vi "updateValues.vi"(8 "error in (no error)":errorcluster, 9 "channel index":i32, 10 "NumberDO":i32, 11 "NumberDI":i32) -> (0 "error out":errorcluster)   [LabVIEW 2020, in "Productivity1000PLC.lvclass"]
uses:
  Productivity1000PLC.lvclass
  shared/OnOffTypeDef.ctl
  shared/CompressAndUpdate(Poly)/CompressAndUpdate(Enum).vi
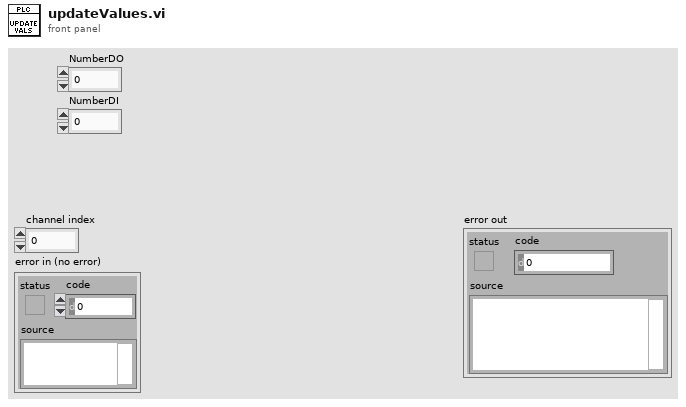
[diagram p1: front panel]
types:
  T1 = typedef "OnOffTypeDef.ctl" = enum16{"off", "on"}
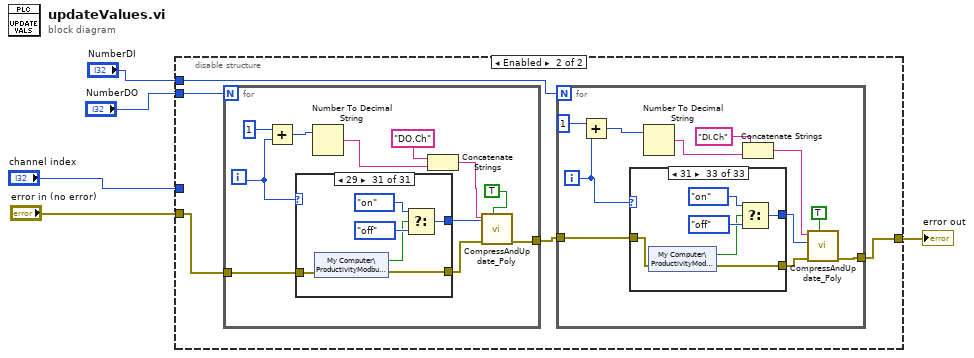
[diagram p0: block diagram]
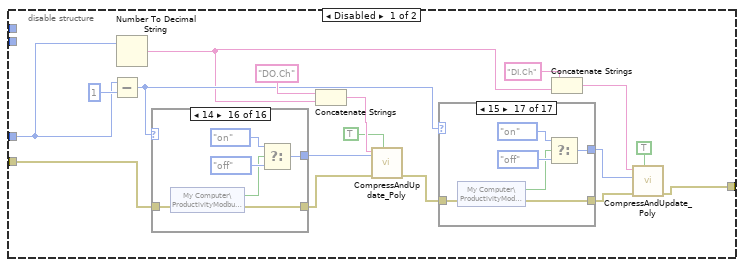
[diagram p2: hidden frame]
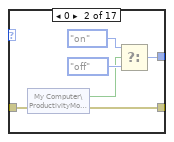
[diagram p4: hidden frame]
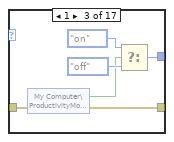
[diagram p5: hidden frame]
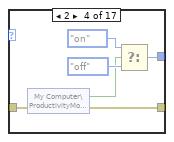
[diagram p6: hidden frame]
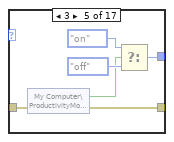
[diagram p7: hidden frame]
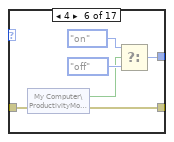
[diagram p8: hidden frame]
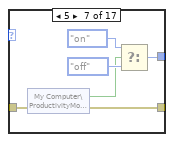
[diagram p9: hidden frame]
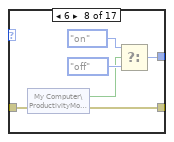
[diagram p10: hidden frame]
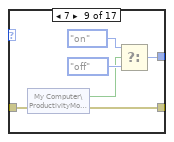
[diagram p11: hidden frame]
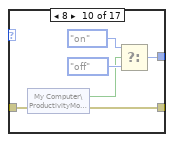
[diagram p12: hidden frame]
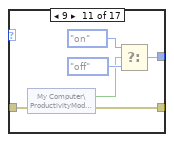
[diagram p13: hidden frame]
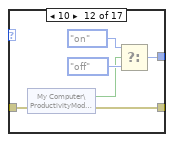
[diagram p14: hidden frame]
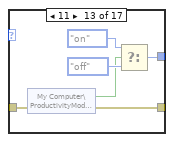
[diagram p15: hidden frame]
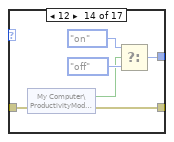
[diagram p16: hidden frame]
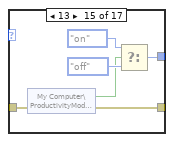
[diagram p17: hidden frame]
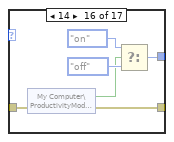
[diagram p18: hidden frame]
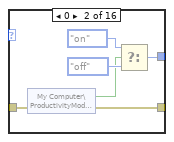
[diagram p20: hidden frame]
diagram:
  n1 = disable-structure shown="Enabled" {
    disable-tunnel: [w15 w213] -> w5
    disable-tunnel: "channel index" -> [w14 _]
    disable-tunnel: "error in (no error)" -> [w13 w215]
    disable-tunnel: "NumberDO" -> [_ w212]
    disable-tunnel: "NumberDI" -> [_ w211]
    frame Disabled {
      n2 = Subtract(x=w14, y=1) -> (x-y=w10:i32)
      n3 = Number To Decimal String(number=w14) -> (decimal integer string=w6:string)  [unwired: 1 in]
      n4 = case shown="14" w10 {
        tunnel: w13 -> [w120 w121 w127 w133 w139 w145 w151 w157 w163 w169 w175 w181 w187 w193 w199 w205]
        tunnel: [w120 w123 w129 w135 w141 w147 w153 w159 w165 w171 w177 w183 w189 w195 w201 w207] -> w9
        tunnel: [_ w122 w128 w134 w140 w146 w152 w158 w164 w170 w176 w182 w188 w194 w200 w206] -> w12
        frame Default {
        }
        frame 0 {
          n5 = shared-variable "My Computer\\ProductivityModbus.lvlib\\DO1"(error in=w121) -> (w124:bool, error out=w123:errorcluster)
          n6 = Select(t=OnOffTypeDef."on" ("Channel 0"), s=w124, f=OnOffTypeDef."off" ("Channel 0")) -> (s? t:f=w122:T1)
        }
        frame 1 {
          n7 = shared-variable "My Computer\\ProductivityModbus.lvlib\\DO2"(error in=w127) -> (w130:bool, error out=w129:errorcluster)
          n8 = Select(t=OnOffTypeDef."on" ("Channel 0"), s=w130, f=OnOffTypeDef."off" ("Channel 0")) -> (s? t:f=w128:T1)
        }
        frame 2 {
          n9 = shared-variable "My Computer\\ProductivityModbus.lvlib\\DO3"(error in=w133) -> (w136:bool, error out=w135:errorcluster)
          n10 = Select(t=OnOffTypeDef."on" ("Channel 0"), s=w136, f=OnOffTypeDef."off" ("Channel 0")) -> (s? t:f=w134:T1)
        }
        frame 3 {
          n11 = shared-variable "My Computer\\ProductivityModbus.lvlib\\DO4"(error in=w139) -> (w142:bool, error out=w141:errorcluster)
          n12 = Select(t=OnOffTypeDef."on" ("Channel 0"), s=w142, f=OnOffTypeDef."off" ("Channel 0")) -> (s? t:f=w140:T1)
        }
        frame 4 {
          n13 = shared-variable "My Computer\\ProductivityModbus.lvlib\\DO5"(error in=w145) -> (w148:bool, error out=w147:errorcluster)
          n14 = Select(t=OnOffTypeDef."on" ("Channel 0"), s=w148, f=OnOffTypeDef."off" ("Channel 0")) -> (s? t:f=w146:T1)
        }
        frame 5 {
          n15 = shared-variable "My Computer\\ProductivityModbus.lvlib\\DO6"(error in=w151) -> (w154:bool, error out=w153:errorcluster)
          n16 = Select(t=OnOffTypeDef."on" ("Channel 0"), s=w154, f=OnOffTypeDef."off" ("Channel 0")) -> (s? t:f=w152:T1)
        }
        frame 6 {
          n17 = shared-variable "My Computer\\ProductivityModbus.lvlib\\DO7"(error in=w157) -> (w160:bool, error out=w159:errorcluster)
          n18 = Select(t=OnOffTypeDef."on" ("Channel 0"), s=w160, f=OnOffTypeDef."off" ("Channel 0")) -> (s? t:f=w158:T1)
        }
        frame 7 {
          n19 = shared-variable "My Computer\\ProductivityModbus.lvlib\\DO8"(error in=w163) -> (w166:bool, error out=w165:errorcluster)
          n20 = Select(t=OnOffTypeDef."on" ("Channel 0"), s=w166, f=OnOffTypeDef."off" ("Channel 0")) -> (s? t:f=w164:T1)
        }
        frame 8 {
          n21 = shared-variable "My Computer\\ProductivityModbus.lvlib\\DO9"(error in=w169) -> (w172:bool, error out=w171:errorcluster)
          n22 = Select(t=OnOffTypeDef."on" ("Channel 0"), s=w172, f=OnOffTypeDef."off" ("Channel 0")) -> (s? t:f=w170:T1)
        }
        frame 9 {
          n23 = shared-variable "My Computer\\ProductivityModbus.lvlib\\DO10"(error in=w175) -> (w178:bool, error out=w177:errorcluster)
          n24 = Select(t=OnOffTypeDef."on" ("Channel 0"), s=w178, f=OnOffTypeDef."off" ("Channel 0")) -> (s? t:f=w176:T1)
        }
        frame 10 {
          n25 = shared-variable "My Computer\\ProductivityModbus.lvlib\\DO11"(error in=w181) -> (w184:bool, error out=w183:errorcluster)
          n26 = Select(t=OnOffTypeDef."on" ("Channel 0"), s=w184, f=OnOffTypeDef."off" ("Channel 0")) -> (s? t:f=w182:T1)
        }
        frame 11 {
          n27 = shared-variable "My Computer\\ProductivityModbus.lvlib\\DO12"(error in=w187) -> (w190:bool, error out=w189:errorcluster)
          n28 = Select(t=OnOffTypeDef."on" ("Channel 0"), s=w190, f=OnOffTypeDef."off" ("Channel 0")) -> (s? t:f=w188:T1)
        }
        frame 12 {
          n29 = shared-variable "My Computer\\ProductivityModbus.lvlib\\DO13"(error in=w193) -> (w196:bool, error out=w195:errorcluster)
          n30 = Select(t=OnOffTypeDef."on" ("Channel 0"), s=w196, f=OnOffTypeDef."off" ("Channel 0")) -> (s? t:f=w194:T1)
        }
        frame 13 {
          n31 = shared-variable "My Computer\\ProductivityModbus.lvlib\\DO14"(error in=w199) -> (w202:bool, error out=w201:errorcluster)
          n32 = Select(t=OnOffTypeDef."on" ("Channel 0"), s=w202, f=OnOffTypeDef."off" ("Channel 0")) -> (s? t:f=w200:T1)
        }
        frame 14 {
          n33 = shared-variable "My Computer\\ProductivityModbus.lvlib\\DO15"(error in=w205) -> (w208:bool, error out=w207:errorcluster)
          n34 = Select(t=OnOffTypeDef."on" ("Channel 0"), s=w208, f=OnOffTypeDef."off" ("Channel 0")) -> (s? t:f=w206:T1)
        }
      }
      n35 = Concatenate Strings("DO.Ch" ("command or variable name"), w6) -> (w22:string)
      n36 = call-poly "CompressAndUpdate_Poly.vi"("force CVT update (false)"=TRUE, "error in"=w9, "enum variant"=w12, "command or variable name"=w22) -> ("error out"=w8:errorcluster)  [unwired: 7 in]
      n37 = case shown="15" w10 {
        tunnel: w8 -> [w23 w24 w30 w36 w42 w48 w54 w60 w66 w72 w78 w84 w90 w96 w102 w108 w114]
        tunnel: [w23 w26 w32 w38 w44 w50 w56 w62 w68 w74 w80 w86 w92 w98 w104 w110 w116] -> w7
        tunnel: [_ w25 w31 w37 w43 w49 w55 w61 w67 w73 w79 w85 w91 w97 w103 w109 w115] -> w11
        frame Default {
        }
        frame 0 {
          n38 = shared-variable "My Computer\\ProductivityModbus.lvlib\\DI1"(error in=w24) -> (w27:bool, error out=w26:errorcluster)
          n39 = Select(t=OnOffTypeDef."on" ("Channel 0"), s=w27, f=OnOffTypeDef."off" ("Channel 0")) -> (s? t:f=w25:T1)
        }
        frame 1 {
          n40 = shared-variable "My Computer\\ProductivityModbus.lvlib\\DI2"(error in=w30) -> (w33:bool, error out=w32:errorcluster)
          n41 = Select(t=OnOffTypeDef."on" ("Channel 0"), s=w33, f=OnOffTypeDef."off" ("Channel 0")) -> (s? t:f=w31:T1)
        }
        frame 2 {
          n42 = shared-variable "My Computer\\ProductivityModbus.lvlib\\DI3"(error in=w36) -> (w39:bool, error out=w38:errorcluster)
          n43 = Select(t=OnOffTypeDef."on" ("Channel 0"), s=w39, f=OnOffTypeDef."off" ("Channel 0")) -> (s? t:f=w37:T1)
        }
        frame 3 {
          n44 = shared-variable "My Computer\\ProductivityModbus.lvlib\\DI4"(error in=w42) -> (w45:bool, error out=w44:errorcluster)
          n45 = Select(t=OnOffTypeDef."on" ("Channel 0"), s=w45, f=OnOffTypeDef."off" ("Channel 0")) -> (s? t:f=w43:T1)
        }
        frame 4 {
          n46 = shared-variable "My Computer\\ProductivityModbus.lvlib\\DI5"(error in=w48) -> (w51:bool, error out=w50:errorcluster)
          n47 = Select(t=OnOffTypeDef."on" ("Channel 0"), s=w51, f=OnOffTypeDef."off" ("Channel 0")) -> (s? t:f=w49:T1)
        }
        frame 5 {
          n48 = shared-variable "My Computer\\ProductivityModbus.lvlib\\DI6"(error in=w54) -> (w57:bool, error out=w56:errorcluster)
          n49 = Select(t=OnOffTypeDef."on" ("Channel 0"), s=w57, f=OnOffTypeDef."off" ("Channel 0")) -> (s? t:f=w55:T1)
        }
        frame 6 {
          n50 = shared-variable "My Computer\\ProductivityModbus.lvlib\\DI7"(error in=w60) -> (w63:bool, error out=w62:errorcluster)
          n51 = Select(t=OnOffTypeDef."on" ("Channel 0"), s=w63, f=OnOffTypeDef."off" ("Channel 0")) -> (s? t:f=w61:T1)
        }
        frame 7 {
          n52 = shared-variable "My Computer\\ProductivityModbus.lvlib\\DI8"(error in=w66) -> (w69:bool, error out=w68:errorcluster)
          n53 = Select(t=OnOffTypeDef."on" ("Channel 0"), s=w69, f=OnOffTypeDef."off" ("Channel 0")) -> (s? t:f=w67:T1)
        }
        frame 8 {
          n54 = shared-variable "My Computer\\ProductivityModbus.lvlib\\DI9"(error in=w72) -> (w75:bool, error out=w74:errorcluster)
          n55 = Select(t=OnOffTypeDef."on" ("Channel 0"), s=w75, f=OnOffTypeDef."off" ("Channel 0")) -> (s? t:f=w73:T1)
        }
        frame 9 {
          n56 = shared-variable "My Computer\\ProductivityModbus.lvlib\\DI10"(error in=w78) -> (w81:bool, error out=w80:errorcluster)
          n57 = Select(t=OnOffTypeDef."on" ("Channel 0"), s=w81, f=OnOffTypeDef."off" ("Channel 0")) -> (s? t:f=w79:T1)
        }
        frame 10 {
          n58 = shared-variable "My Computer\\ProductivityModbus.lvlib\\DI11"(error in=w84) -> (w87:bool, error out=w86:errorcluster)
          n59 = Select(t=OnOffTypeDef."on" ("Channel 0"), s=w87, f=OnOffTypeDef."off" ("Channel 0")) -> (s? t:f=w85:T1)
        }
        frame 11 {
          n60 = shared-variable "My Computer\\ProductivityModbus.lvlib\\DI12"(error in=w90) -> (w93:bool, error out=w92:errorcluster)
          n61 = Select(t=OnOffTypeDef."on" ("Channel 0"), s=w93, f=OnOffTypeDef."off" ("Channel 0")) -> (s? t:f=w91:T1)
        }
        frame 12 {
          n62 = shared-variable "My Computer\\ProductivityModbus.lvlib\\DI13"(error in=w96) -> (w99:bool, error out=w98:errorcluster)
          n63 = Select(t=OnOffTypeDef."on" ("Channel 0"), s=w99, f=OnOffTypeDef."off" ("Channel 0")) -> (s? t:f=w97:T1)
        }
        frame 13 {
          n64 = shared-variable "My Computer\\ProductivityModbus.lvlib\\DI14"(error in=w102) -> (w105:bool, error out=w104:errorcluster)
          n65 = Select(t=OnOffTypeDef."on" ("Channel 0"), s=w105, f=OnOffTypeDef."off" ("Channel 0")) -> (s? t:f=w103:T1)
        }
        frame 14 {
          n66 = shared-variable "My Computer\\ProductivityModbus.lvlib\\DI15"(error in=w108) -> (w111:bool, error out=w110:errorcluster)
          n67 = Select(t=OnOffTypeDef."on" ("Channel 0"), s=w111, f=OnOffTypeDef."off" ("Channel 0")) -> (s? t:f=w109:T1)
        }
        frame 15 {
          n68 = shared-variable "My Computer\\ProductivityModbus.lvlib\\DI16"(error in=w114) -> (w117:bool, error out=w116:errorcluster)
          n69 = Select(t=OnOffTypeDef."on" ("Channel 0"), s=w117, f=OnOffTypeDef."off" ("Channel 0")) -> (s? t:f=w115:T1)
        }
      }
      n70 = Concatenate Strings("DI.Ch" ("command or variable name"), w6) -> (w18:string)
      n71 = call-poly "CompressAndUpdate_Poly.vi"("force CVT update (false)"=TRUE, "error in"=w7, "enum variant"=w11, "command or variable name"=w18) -> ("error out"=w15:errorcluster)  [unwired: 7 in]
    }
    frame Enabled {
      n72 = for {
        N: w212 -> [_]
        tunnel: w215 -> [w424]
        tunnel: [w423] -> w214
        i -> [w422]
        n73 = Add(x=1, y=w422) -> (x+y=w420:i32)
        n74 = case shown="29" w422 {
          tunnel: [w431 w434 w440 w446 w452 w458 w464 w470 w476 w482 w488 w494 w500 w506 w512 w518 w524 w530 w536 w542 w548 w554 w560 w566 w572 w578 w584 w590 w596 w602 w608] -> w426
          tunnel: [_ w433 w439 w445 w451 w457 w463 w469 w475 w481 w487 w493 w499 w505 w511 w517 w523 w529 w535 w541 w547 w553 w559 w565 w571 w577 w583 w589 w595 w601 w607] -> w427
          tunnel: w424 -> [w431 w432 w438 w444 w450 w456 w462 w468 w474 w480 w486 w492 w498 w504 w510 w516 w522 w528 w534 w540 w546 w552 w558 w564 w570 w576 w582 w588 w594 w600 w606]
          frame Default {
          }
          frame 0 {
            n75 = shared-variable "My Computer\\ProductivityModbus.lvlib\\DO1"(error in=w432) -> (w435:bool, error out=w434:errorcluster)
            n76 = Select(t=OnOffTypeDef."on" ("Channel 0"), s=w435, f=OnOffTypeDef."off" ("Channel 0")) -> (s? t:f=w433:T1)
          }
          frame 1 {
            n77 = shared-variable "My Computer\\ProductivityModbus.lvlib\\DO2"(error in=w438) -> (w441:bool, error out=w440:errorcluster)
            n78 = Select(t=OnOffTypeDef."on" ("Channel 0"), s=w441, f=OnOffTypeDef."off" ("Channel 0")) -> (s? t:f=w439:T1)
          }
          frame 2 {
            n79 = shared-variable "My Computer\\ProductivityModbus.lvlib\\DO3"(error in=w444) -> (w447:bool, error out=w446:errorcluster)
            n80 = Select(t=OnOffTypeDef."on" ("Channel 0"), s=w447, f=OnOffTypeDef."off" ("Channel 0")) -> (s? t:f=w445:T1)
          }
          frame 3 {
            n81 = shared-variable "My Computer\\ProductivityModbus.lvlib\\DO4"(error in=w450) -> (w453:bool, error out=w452:errorcluster)
            n82 = Select(t=OnOffTypeDef."on" ("Channel 0"), s=w453, f=OnOffTypeDef."off" ("Channel 0")) -> (s? t:f=w451:T1)
          }
          frame 4 {
            n83 = shared-variable "My Computer\\ProductivityModbus.lvlib\\DO5"(error in=w456) -> (w459:bool, error out=w458:errorcluster)
            n84 = Select(t=OnOffTypeDef."on" ("Channel 0"), s=w459, f=OnOffTypeDef."off" ("Channel 0")) -> (s? t:f=w457:T1)
          }
          frame 5 {
            n85 = shared-variable "My Computer\\ProductivityModbus.lvlib\\DO6"(error in=w462) -> (w465:bool, error out=w464:errorcluster)
            n86 = Select(t=OnOffTypeDef."on" ("Channel 0"), s=w465, f=OnOffTypeDef."off" ("Channel 0")) -> (s? t:f=w463:T1)
          }
          frame 6 {
            n87 = shared-variable "My Computer\\ProductivityModbus.lvlib\\DO7"(error in=w468) -> (w471:bool, error out=w470:errorcluster)
            n88 = Select(t=OnOffTypeDef."on" ("Channel 0"), s=w471, f=OnOffTypeDef."off" ("Channel 0")) -> (s? t:f=w469:T1)
          }
          frame 7 {
            n89 = shared-variable "My Computer\\ProductivityModbus.lvlib\\DO8"(error in=w474) -> (w477:bool, error out=w476:errorcluster)
            n90 = Select(t=OnOffTypeDef."on" ("Channel 0"), s=w477, f=OnOffTypeDef."off" ("Channel 0")) -> (s? t:f=w475:T1)
          }
          frame 8 {
            n91 = shared-variable "My Computer\\ProductivityModbus.lvlib\\DO9"(error in=w480) -> (w483:bool, error out=w482:errorcluster)
            n92 = Select(t=OnOffTypeDef."on" ("Channel 0"), s=w483, f=OnOffTypeDef."off" ("Channel 0")) -> (s? t:f=w481:T1)
          }
          frame 9 {
            n93 = shared-variable "My Computer\\ProductivityModbus.lvlib\\DO10"(error in=w486) -> (w489:bool, error out=w488:errorcluster)
            n94 = Select(t=OnOffTypeDef."on" ("Channel 0"), s=w489, f=OnOffTypeDef."off" ("Channel 0")) -> (s? t:f=w487:T1)
          }
          frame 10 {
            n95 = shared-variable "My Computer\\ProductivityModbus.lvlib\\DO11"(error in=w492) -> (w495:bool, error out=w494:errorcluster)
            n96 = Select(t=OnOffTypeDef."on" ("Channel 0"), s=w495, f=OnOffTypeDef."off" ("Channel 0")) -> (s? t:f=w493:T1)
          }
          frame 11 {
            n97 = shared-variable "My Computer\\ProductivityModbus.lvlib\\DO12"(error in=w498) -> (w501:bool, error out=w500:errorcluster)
            n98 = Select(t=OnOffTypeDef."on" ("Channel 0"), s=w501, f=OnOffTypeDef."off" ("Channel 0")) -> (s? t:f=w499:T1)
          }
          frame 12 {
            n99 = shared-variable "My Computer\\ProductivityModbus.lvlib\\DO13"(error in=w504) -> (w507:bool, error out=w506:errorcluster)
            n100 = Select(t=OnOffTypeDef."on" ("Channel 0"), s=w507, f=OnOffTypeDef."off" ("Channel 0")) -> (s? t:f=w505:T1)
          }
          frame 13 {
            n101 = shared-variable "My Computer\\ProductivityModbus.lvlib\\DO14"(error in=w510) -> (w513:bool, error out=w512:errorcluster)
            n102 = Select(t=OnOffTypeDef."on" ("Channel 0"), s=w513, f=OnOffTypeDef."off" ("Channel 0")) -> (s? t:f=w511:T1)
          }
          frame 14 {
            n103 = shared-variable "My Computer\\ProductivityModbus.lvlib\\DO15"(error in=w516) -> (w519:bool, error out=w518:errorcluster)
            n104 = Select(t=OnOffTypeDef."on" ("Channel 0"), s=w519, f=OnOffTypeDef."off" ("Channel 0")) -> (s? t:f=w517:T1)
          }
          frame 15 {
            n105 = shared-variable "My Computer\\ProductivityModbus.lvlib\\DO16"(error in=w522) -> (w525:bool, error out=w524:errorcluster)
            n106 = Select(t=OnOffTypeDef."on" ("Channel 0"), s=w525, f=OnOffTypeDef."off" ("Channel 0")) -> (s? t:f=w523:T1)
          }
          frame 16 {
            n107 = shared-variable "My Computer\\ProductivityModbus.lvlib\\DO17"(error in=w528) -> (w531:bool, error out=w530:errorcluster)
            n108 = Select(t=OnOffTypeDef."on" ("Channel 0"), s=w531, f=OnOffTypeDef."off" ("Channel 0")) -> (s? t:f=w529:T1)
          }
          frame 17 {
            n109 = shared-variable "My Computer\\ProductivityModbus.lvlib\\DO18"(error in=w534) -> (w537:bool, error out=w536:errorcluster)
            n110 = Select(t=OnOffTypeDef."on" ("Channel 0"), s=w537, f=OnOffTypeDef."off" ("Channel 0")) -> (s? t:f=w535:T1)
          }
          frame 18 {
            n111 = shared-variable "My Computer\\ProductivityModbus.lvlib\\DO19"(error in=w540) -> (w543:bool, error out=w542:errorcluster)
            n112 = Select(t=OnOffTypeDef."on" ("Channel 0"), s=w543, f=OnOffTypeDef."off" ("Channel 0")) -> (s? t:f=w541:T1)
          }
          frame 19 {
            n113 = shared-variable "My Computer\\ProductivityModbus.lvlib\\DO20"(error in=w546) -> (w549:bool, error out=w548:errorcluster)
            n114 = Select(t=OnOffTypeDef."on" ("Channel 0"), s=w549, f=OnOffTypeDef."off" ("Channel 0")) -> (s? t:f=w547:T1)
          }
          frame 20 {
            n115 = shared-variable "My Computer\\ProductivityModbus.lvlib\\DO21"(error in=w552) -> (w555:bool, error out=w554:errorcluster)
            n116 = Select(t=OnOffTypeDef."on" ("Channel 0"), s=w555, f=OnOffTypeDef."off" ("Channel 0")) -> (s? t:f=w553:T1)
          }
          frame 21 {
            n117 = shared-variable "My Computer\\ProductivityModbus.lvlib\\DO22"(error in=w558) -> (w561:bool, error out=w560:errorcluster)
            n118 = Select(t=OnOffTypeDef."on" ("Channel 0"), s=w561, f=OnOffTypeDef."off" ("Channel 0")) -> (s? t:f=w559:T1)
          }
          frame 22 {
            n119 = shared-variable "My Computer\\ProductivityModbus.lvlib\\DO23"(error in=w564) -> (w567:bool, error out=w566:errorcluster)
            n120 = Select(t=OnOffTypeDef."on" ("Channel 0"), s=w567, f=OnOffTypeDef."off" ("Channel 0")) -> (s? t:f=w565:T1)
          }
          frame 23 {
            n121 = shared-variable "My Computer\\ProductivityModbus.lvlib\\DO24"(error in=w570) -> (w573:bool, error out=w572:errorcluster)
            n122 = Select(t=OnOffTypeDef."on" ("Channel 0"), s=w573, f=OnOffTypeDef."off" ("Channel 0")) -> (s? t:f=w571:T1)
          }
          frame 24 {
            n123 = shared-variable "My Computer\\ProductivityModbus.lvlib\\DO25"(error in=w576) -> (w579:bool, error out=w578:errorcluster)
            n124 = Select(t=OnOffTypeDef."on" ("Channel 0"), s=w579, f=OnOffTypeDef."off" ("Channel 0")) -> (s? t:f=w577:T1)
          }
          frame 25 {
            n125 = shared-variable "My Computer\\ProductivityModbus.lvlib\\DO26"(error in=w582) -> (w585:bool, error out=w584:errorcluster)
            n126 = Select(t=OnOffTypeDef."on" ("Channel 0"), s=w585, f=OnOffTypeDef."off" ("Channel 0")) -> (s? t:f=w583:T1)
          }
          frame 26 {
            n127 = shared-variable "My Computer\\ProductivityModbus.lvlib\\DO27"(error in=w588) -> (w591:bool, error out=w590:errorcluster)
            n128 = Select(t=OnOffTypeDef."on" ("Channel 0"), s=w591, f=OnOffTypeDef."off" ("Channel 0")) -> (s? t:f=w589:T1)
          }
          frame 27 {
            n129 = shared-variable "My Computer\\ProductivityModbus.lvlib\\DO28"(error in=w594) -> (w597:bool, error out=w596:errorcluster)
            n130 = Select(t=OnOffTypeDef."on" ("Channel 0"), s=w597, f=OnOffTypeDef."off" ("Channel 0")) -> (s? t:f=w595:T1)
          }
          frame 28 {
            n131 = shared-variable "My Computer\\ProductivityModbus.lvlib\\DO29"(error in=w600) -> (w603:bool, error out=w602:errorcluster)
            n132 = Select(t=OnOffTypeDef."on" ("Channel 0"), s=w603, f=OnOffTypeDef."off" ("Channel 0")) -> (s? t:f=w601:T1)
          }
          frame 29 {
            n133 = shared-variable "My Computer\\ProductivityModbus.lvlib\\DO30"(error in=w606) -> (w609:bool, error out=w608:errorcluster)
            n134 = Select(t=OnOffTypeDef."on" ("Channel 0"), s=w609, f=OnOffTypeDef."off" ("Channel 0")) -> (s? t:f=w607:T1)
          }
        }
        n135 = Number To Decimal String(number=w420) -> (decimal integer string=w425:string)  [unwired: 1 in]
        n136 = Concatenate Strings("DO.Ch" ("command or variable name"), w425) -> (w430:string)
        n137 = call-poly "CompressAndUpdate_Poly.vi"("force CVT update (false)"=TRUE, "error in"=w426, "enum variant"=w427, "command or variable name"=w430) -> ("error out"=w423:errorcluster)  [unwired: 7 in]
      }
      n138 = for {
        N: w211 -> [_]
        tunnel: [w220] -> w213
        tunnel: w214 -> [w219]
        i -> [w216]
        n139 = Add(x=1, y=w216) -> (x+y=w217:i32)
        n140 = case shown="31" w216 {
          tunnel: [w227 w230 w236 w242 w248 w254 w260 w266 w272 w278 w284 w290 w296 w302 w308 w314 w320 w326 w332 w338 w344 w350 w356 w362 w368 w374 w380 w386 w392 w398 w404 w410 w416] -> w222
          tunnel: [_ w229 w235 w241 w247 w253 w259 w265 w271 w277 w283 w289 w295 w301 w307 w313 w319 w325 w331 w337 w343 w349 w355 w361 w367 w373 w379 w385 w391 w397 w403 w409 w415] -> w223
          tunnel: w219 -> [w227 w228 w234 w240 w246 w252 w258 w264 w270 w276 w282 w288 w294 w300 w306 w312 w318 w324 w330 w336 w342 w348 w354 w360 w366 w372 w378 w384 w390 w396 w402 w408 w414]
          frame Default {
          }
          frame 0 {
            n141 = shared-variable "My Computer\\ProductivityModbus.lvlib\\DI1"(error in=w228) -> (w231:bool, error out=w230:errorcluster)
            n142 = Select(t=OnOffTypeDef."on" ("Channel 0"), s=w231, f=OnOffTypeDef."off" ("Channel 0")) -> (s? t:f=w229:T1)
          }
          frame 1 {
            n143 = shared-variable "My Computer\\ProductivityModbus.lvlib\\DI2"(error in=w234) -> (w237:bool, error out=w236:errorcluster)
            n144 = Select(t=OnOffTypeDef."on" ("Channel 0"), s=w237, f=OnOffTypeDef."off" ("Channel 0")) -> (s? t:f=w235:T1)
          }
          frame 2 {
            n145 = shared-variable "My Computer\\ProductivityModbus.lvlib\\DI3"(error in=w240) -> (w243:bool, error out=w242:errorcluster)
            n146 = Select(t=OnOffTypeDef."on" ("Channel 0"), s=w243, f=OnOffTypeDef."off" ("Channel 0")) -> (s? t:f=w241:T1)
          }
          frame 3 {
            n147 = shared-variable "My Computer\\ProductivityModbus.lvlib\\DI4"(error in=w246) -> (w249:bool, error out=w248:errorcluster)
            n148 = Select(t=OnOffTypeDef."on" ("Channel 0"), s=w249, f=OnOffTypeDef."off" ("Channel 0")) -> (s? t:f=w247:T1)
          }
          frame 4 {
            n149 = shared-variable "My Computer\\ProductivityModbus.lvlib\\DI5"(error in=w252) -> (w255:bool, error out=w254:errorcluster)
            n150 = Select(t=OnOffTypeDef."on" ("Channel 0"), s=w255, f=OnOffTypeDef."off" ("Channel 0")) -> (s? t:f=w253:T1)
          }
          frame 5 {
            n151 = shared-variable "My Computer\\ProductivityModbus.lvlib\\DI6"(error in=w258) -> (w261:bool, error out=w260:errorcluster)
            n152 = Select(t=OnOffTypeDef."on" ("Channel 0"), s=w261, f=OnOffTypeDef."off" ("Channel 0")) -> (s? t:f=w259:T1)
          }
          frame 6 {
            n153 = shared-variable "My Computer\\ProductivityModbus.lvlib\\DI7"(error in=w264) -> (w267:bool, error out=w266:errorcluster)
            n154 = Select(t=OnOffTypeDef."on" ("Channel 0"), s=w267, f=OnOffTypeDef."off" ("Channel 0")) -> (s? t:f=w265:T1)
          }
          frame 7 {
            n155 = shared-variable "My Computer\\ProductivityModbus.lvlib\\DI8"(error in=w270) -> (w273:bool, error out=w272:errorcluster)
            n156 = Select(t=OnOffTypeDef."on" ("Channel 0"), s=w273, f=OnOffTypeDef."off" ("Channel 0")) -> (s? t:f=w271:T1)
          }
          frame 8 {
            n157 = shared-variable "My Computer\\ProductivityModbus.lvlib\\DI9"(error in=w276) -> (w279:bool, error out=w278:errorcluster)
            n158 = Select(t=OnOffTypeDef."on" ("Channel 0"), s=w279, f=OnOffTypeDef."off" ("Channel 0")) -> (s? t:f=w277:T1)
          }
          frame 9 {
            n159 = shared-variable "My Computer\\ProductivityModbus.lvlib\\DI10"(error in=w282) -> (w285:bool, error out=w284:errorcluster)
            n160 = Select(t=OnOffTypeDef."on" ("Channel 0"), s=w285, f=OnOffTypeDef."off" ("Channel 0")) -> (s? t:f=w283:T1)
          }
          frame 10 {
            n161 = shared-variable "My Computer\\ProductivityModbus.lvlib\\DI11"(error in=w288) -> (w291:bool, error out=w290:errorcluster)
            n162 = Select(t=OnOffTypeDef."on" ("Channel 0"), s=w291, f=OnOffTypeDef."off" ("Channel 0")) -> (s? t:f=w289:T1)
          }
          frame 11 {
            n163 = shared-variable "My Computer\\ProductivityModbus.lvlib\\DI12"(error in=w294) -> (w297:bool, error out=w296:errorcluster)
            n164 = Select(t=OnOffTypeDef."on" ("Channel 0"), s=w297, f=OnOffTypeDef."off" ("Channel 0")) -> (s? t:f=w295:T1)
          }
          frame 12 {
            n165 = shared-variable "My Computer\\ProductivityModbus.lvlib\\DI13"(error in=w300) -> (w303:bool, error out=w302:errorcluster)
            n166 = Select(t=OnOffTypeDef."on" ("Channel 0"), s=w303, f=OnOffTypeDef."off" ("Channel 0")) -> (s? t:f=w301:T1)
          }
          frame 13 {
            n167 = shared-variable "My Computer\\ProductivityModbus.lvlib\\DI14"(error in=w306) -> (w309:bool, error out=w308:errorcluster)
            n168 = Select(t=OnOffTypeDef."on" ("Channel 0"), s=w309, f=OnOffTypeDef."off" ("Channel 0")) -> (s? t:f=w307:T1)
          }
          frame 14 {
            n169 = shared-variable "My Computer\\ProductivityModbus.lvlib\\DI15"(error in=w312) -> (w315:bool, error out=w314:errorcluster)
            n170 = Select(t=OnOffTypeDef."on" ("Channel 0"), s=w315, f=OnOffTypeDef."off" ("Channel 0")) -> (s? t:f=w313:T1)
          }
          frame 15 {
            n171 = shared-variable "My Computer\\ProductivityModbus.lvlib\\DI16"(error in=w318) -> (w321:bool, error out=w320:errorcluster)
            n172 = Select(t=OnOffTypeDef."on" ("Channel 0"), s=w321, f=OnOffTypeDef."off" ("Channel 0")) -> (s? t:f=w319:T1)
          }
          frame 16 {
            n173 = shared-variable "My Computer\\ProductivityModbus.lvlib\\DI17"(error in=w324) -> (w327:bool, error out=w326:errorcluster)
            n174 = Select(t=OnOffTypeDef."on" ("Channel 0"), s=w327, f=OnOffTypeDef."off" ("Channel 0")) -> (s? t:f=w325:T1)
          }
          frame 17 {
            n175 = shared-variable "My Computer\\ProductivityModbus.lvlib\\DI18"(error in=w330) -> (w333:bool, error out=w332:errorcluster)
            n176 = Select(t=OnOffTypeDef."on" ("Channel 0"), s=w333, f=OnOffTypeDef."off" ("Channel 0")) -> (s? t:f=w331:T1)
          }
          frame 18 {
            n177 = shared-variable "My Computer\\ProductivityModbus.lvlib\\DI19"(error in=w336) -> (w339:bool, error out=w338:errorcluster)
            n178 = Select(t=OnOffTypeDef."on" ("Channel 0"), s=w339, f=OnOffTypeDef."off" ("Channel 0")) -> (s? t:f=w337:T1)
          }
          frame 19 {
            n179 = shared-variable "My Computer\\ProductivityModbus.lvlib\\DI20"(error in=w342) -> (w345:bool, error out=w344:errorcluster)
            n180 = Select(t=OnOffTypeDef."on" ("Channel 0"), s=w345, f=OnOffTypeDef."off" ("Channel 0")) -> (s? t:f=w343:T1)
          }
          frame 20 {
            n181 = shared-variable "My Computer\\ProductivityModbus.lvlib\\DI21"(error in=w348) -> (w351:bool, error out=w350:errorcluster)
            n182 = Select(t=OnOffTypeDef."on" ("Channel 0"), s=w351, f=OnOffTypeDef."off" ("Channel 0")) -> (s? t:f=w349:T1)
          }
          frame 21 {
            n183 = shared-variable "My Computer\\ProductivityModbus.lvlib\\DI22"(error in=w354) -> (w357:bool, error out=w356:errorcluster)
            n184 = Select(t=OnOffTypeDef."on" ("Channel 0"), s=w357, f=OnOffTypeDef."off" ("Channel 0")) -> (s? t:f=w355:T1)
          }
          frame 22 {
            n185 = shared-variable "My Computer\\ProductivityModbus.lvlib\\DI23"(error in=w360) -> (w363:bool, error out=w362:errorcluster)
            n186 = Select(t=OnOffTypeDef."on" ("Channel 0"), s=w363, f=OnOffTypeDef."off" ("Channel 0")) -> (s? t:f=w361:T1)
          }
          frame 23 {
            n187 = shared-variable "My Computer\\ProductivityModbus.lvlib\\DI24"(error in=w366) -> (w369:bool, error out=w368:errorcluster)
            n188 = Select(t=OnOffTypeDef."on" ("Channel 0"), s=w369, f=OnOffTypeDef."off" ("Channel 0")) -> (s? t:f=w367:T1)
          }
          frame 24 {
            n189 = shared-variable "My Computer\\ProductivityModbus.lvlib\\DI25"(error in=w372) -> (w375:bool, error out=w374:errorcluster)
            n190 = Select(t=OnOffTypeDef."on" ("Channel 0"), s=w375, f=OnOffTypeDef."off" ("Channel 0")) -> (s? t:f=w373:T1)
          }
          frame 25 {
            n191 = shared-variable "My Computer\\ProductivityModbus.lvlib\\DI26"(error in=w378) -> (w381:bool, error out=w380:errorcluster)
            n192 = Select(t=OnOffTypeDef."on" ("Channel 0"), s=w381, f=OnOffTypeDef."off" ("Channel 0")) -> (s? t:f=w379:T1)
          }
          frame 26 {
            n193 = shared-variable "My Computer\\ProductivityModbus.lvlib\\DI27"(error in=w384) -> (w387:bool, error out=w386:errorcluster)
            n194 = Select(t=OnOffTypeDef."on" ("Channel 0"), s=w387, f=OnOffTypeDef."off" ("Channel 0")) -> (s? t:f=w385:T1)
          }
          frame 27 {
            n195 = shared-variable "My Computer\\ProductivityModbus.lvlib\\DI28"(error in=w390) -> (w393:bool, error out=w392:errorcluster)
            n196 = Select(t=OnOffTypeDef."on" ("Channel 0"), s=w393, f=OnOffTypeDef."off" ("Channel 0")) -> (s? t:f=w391:T1)
          }
          frame 28 {
            n197 = shared-variable "My Computer\\ProductivityModbus.lvlib\\DI29"(error in=w396) -> (w399:bool, error out=w398:errorcluster)
            n198 = Select(t=OnOffTypeDef."on" ("Channel 0"), s=w399, f=OnOffTypeDef."off" ("Channel 0")) -> (s? t:f=w397:T1)
          }
          frame 29 {
            n199 = shared-variable "My Computer\\ProductivityModbus.lvlib\\DI30"(error in=w402) -> (w405:bool, error out=w404:errorcluster)
            n200 = Select(t=OnOffTypeDef."on" ("Channel 0"), s=w405, f=OnOffTypeDef."off" ("Channel 0")) -> (s? t:f=w403:T1)
          }
          frame 30 {
            n201 = shared-variable "My Computer\\ProductivityModbus.lvlib\\DI31"(error in=w408) -> (w411:bool, error out=w410:errorcluster)
            n202 = Select(t=OnOffTypeDef."on" ("Channel 0"), s=w411, f=OnOffTypeDef."off" ("Channel 0")) -> (s? t:f=w409:T1)
          }
          frame 31 {
            n203 = shared-variable "My Computer\\ProductivityModbus.lvlib\\DI32"(error in=w414) -> (w417:bool, error out=w416:errorcluster)
            n204 = Select(t=OnOffTypeDef."on" ("Channel 0"), s=w417, f=OnOffTypeDef."off" ("Channel 0")) -> (s? t:f=w415:T1)
          }
        }
        n205 = Number To Decimal String(number=w217) -> (decimal integer string=w221:string)  [unwired: 1 in]
        n206 = Concatenate Strings("DI.Ch" ("command or variable name"), w221) -> (w226:string)
        n207 = call-poly "CompressAndUpdate_Poly.vi"("force CVT update (false)"=TRUE, "error in"=w222, "enum variant"=w223, "command or variable name"=w226) -> ("error out"=w220:errorcluster)  [unwired: 7 in]
      }
    }
  }
  "error out" <- w5
